vi "GEOM_GetWCSOverride_data.vi"(9 "override headers":string[][](array[string]), 10 "sheaders in":string[][](array[string])) -> (2 "sheaders out":string[][](array[string]))   [LabVIEW 2016]
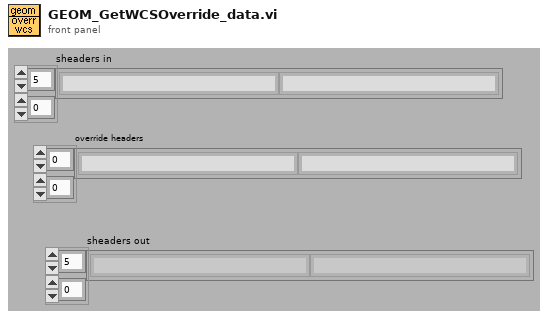
[diagram p1: front panel]
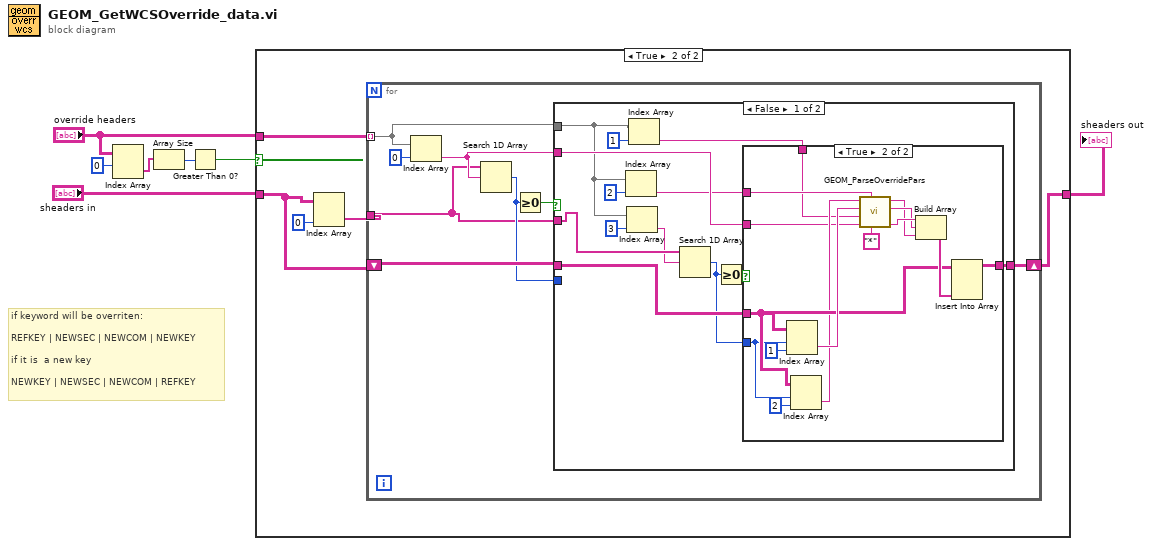
[diagram p0: block diagram]
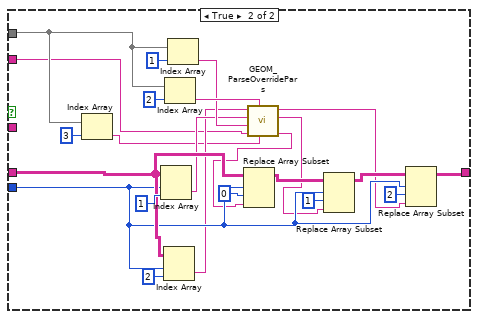
[diagram p4: hidden frame]
diagram:
  # "if keyword will be overriten:\n\nREFKEY | NEWSEC | NEWCOM | NEWKEY\n\nif it is  a new key\n\nNEWKEY | NEWSEC | NEWCOM | REFKEY"
  n1 = Index Array(array="override headers", index (col)=0 ("disabled index (col)")) -> (element=w1:string[])  [unwired: 1 in]
  n2 = Array Size(array=w1) -> (size(s)=w7:i32)
  n3 = Greater Than 0?(x=w7) -> (x > 0?=w6:bool)
  n4 = case shown="True" w6 {
    tunnel: "override headers" -> [_ w13]
    tunnel: "sheaders in" -> [w8 w10]
    tunnel: [w8 w9] -> w4
    frame False {
    }
    frame True {
      n5 = Index Array(array=w10, index (col)=0 ("disabled index (col)")) -> (element=w11:string[])  [unwired: 1 in]
      n6 = for {
        tunnel: w13 -> [w17] mode=indexing
        shift-right: [w18] -> w9
        shift-left: w10 -> [w19]
        tunnel: w11 -> [w14]
        n7 = Index Array(array=w17, index=0) -> (element=w15:string)
        n8 = Search 1D Array(1D array=w14, element=w15) -> (index of element=w16:i32)  [unwired: 1 out]
        n9 = Greater Or Equal To 0?(x=w16) -> (x >= 0?=w20:bool)
        n10 = case shown="False" w20 {
          tunnel: w19 -> [w30 w61]
          tunnel: [w29 w67] -> w18
          tunnel: w17 -> [w25 w64]
          tunnel: w16 -> [_ w60]
          tunnel: w15 -> [w27 w54]
          tunnel: w14 -> [w33 _]
          frame False {
            n11 = Index Array(array=w25, index=2) -> (element=w23:string)
            n12 = Index Array(array=w25, index=3) -> (element=w32:string)
            n13 = Index Array(array=w25, index=1) -> (element=w22:string)
            n14 = Search 1D Array(1D array=w33, element=w32) -> (index of element=w28:i32)  [unwired: 1 out]
            n15 = Greater Or Equal To 0?(x=w28) -> (x >= 0?=w31:bool)
            n16 = case shown="True" w31 {
              tunnel: w30 -> [w35 w43]
              tunnel: [w35 w50] -> w29
              tunnel: w28 -> [_ w42]
              tunnel: w27 -> [_ w39]
              tunnel: w23 -> [_ w37]
              tunnel: w22 -> [_ w36]
              frame False {
              }
              frame True {
                n17 = Index Array(array=w43, index (row)=w42, index (col)=1 ("disabled index (col)")) -> (element=w44:string)
                n18 = Index Array(array=w43, index (row)=w42, index (col)=2 ("disabled index (col)")) -> (element=w40:string)
                n19 = call "GEOM_ParseOverridePars.vi"("override keyword"="*", "override comment"=w37, "keyword in"=w39, "override pars"=w36, "section in"=w44, "comment in"=w40) -> ("keyword out"=w49:string, "section out"=w48:string, "comment out"=w47:string)  [unwired: 3 out]
                n20 = Build Array(w49, w48, w47) -> (w46:string[])
                n21 = Insert Into Array(array=w43, new element=w46) -> (w50:string[][])  [unwired: 2 in]
              }
            }
          }
          frame True {
            n22 = Index Array(array=w64, index=3) -> (element=w55:string)
            n23 = Index Array(array=w61, index (row)=w60, index (col)=1 ("index")) -> (element=w57:string)
            n24 = Index Array(array=w61, index (row)=w60, index (col)=2 ("disabled index (col)")) -> (element=w56:string)
            n25 = Index Array(array=w64, index=2) -> (element=w59:string)
            n26 = Index Array(array=w64, index=1) -> (element=w58:string)
            n27 = call "GEOM_ParseOverridePars.vi"("override keyword"=w55, "override comment"=w59, "keyword in"=w54, "override pars"=w58, "section in"=w57, "comment in"=w56) -> ("keyword out"=w53:string, "section out"=w52:string, "comment out"=w51:string)  [unwired: 3 out]
            n28 = Replace Array Subset(array=w61, new element=w53, index (row)=w60, index (col)=0 ("disabled index (col)")) -> (w63:string[][])
            n29 = Replace Array Subset(array=w63, new element=w52, index (row)=w60, index (col)=1 ("disabled index (col)")) -> (w68:string[][])
            n30 = Replace Array Subset(array=w68, new element=w51, index (row)=w60, index (col)=2 ("disabled index (col)")) -> (w67:string[][])
          }
        }
      }
    }
  }
  "sheaders out" <- w4
